vi "Plot Data - Main GUI.vi"() -> ()   [LabVIEW 2017, in "DTacq Plot Display Library.lvlib"]
doc: "This VI is used to display data from the DTacq network enabled drivers.\n\nClicking settings allows the plots on the current tab to be configured."
uses:
  DTacq Plot Display Library.lvlib
  Typedefs/Program Commands--Enum.ctl
  Typedefs/Plot Channel Configruation--Cluster.ctl
  SubVIs/Plot Data--Cluster.ctl
  Network Shared Variables/Typedefs/X and Y Variant Arrays--Cluster.ctl
  Typedefs/Graphical Interface Commands - Tabs--Enum.ctl
  Typedefs/Graphical Interface Commands - Plot--Enum.ctl
  Network Shared Variables/Shared Variables Library.lvlib
panel:
  out "Activity":bool
  out "Last Update":timestamp
  in  "Close Tab Button":bool
  out "XY Plot Title":string
  in  "Add Tab Button":bool
  out "XY Graph":cluster{i32[], i32[]}[](graph)
  in  "Tab Control":T1(tab)
  in  "Save Button":bool
  in  "Settings Button":bool
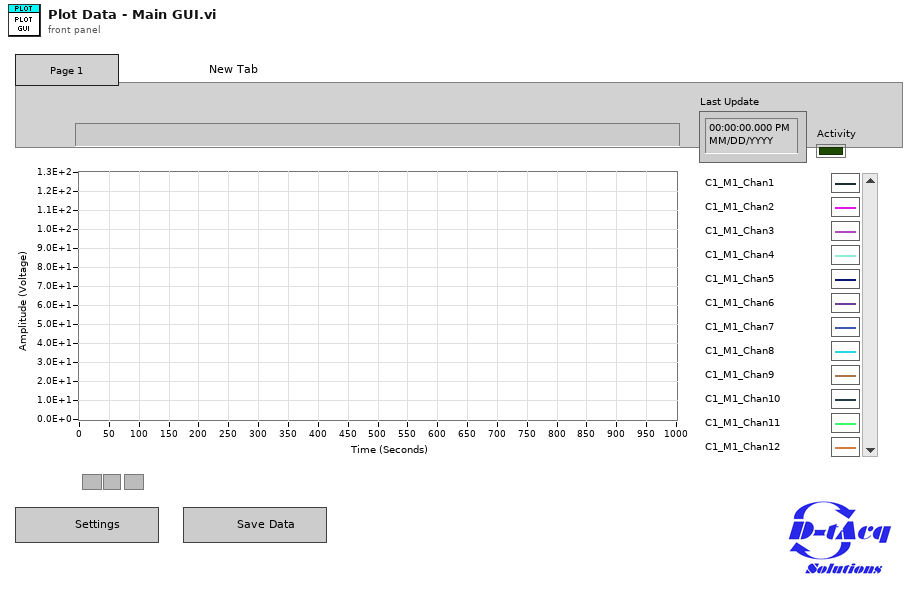
[diagram p1: front panel]
types:
  T1 = enum32{"Page 1", "Page 2", "Page 3", "Page 4", "Page 5", "Page 6"}
  T2 = typedef "DTacq Plot Display Library.lvlib/Plot Data--Cluster.ctl" = cluster{"Last Update":timestamp, "Data Cluster":T3}
  T3 = typedef "Shared Variables Library.lvlib/X and Y Variant Arrays--Cluster.ctl" = cluster{"X-Data":variant[], "Y-Data":variant[]}
  T4 = typedef "DTacq Plot Display Library.lvlib/Plot Channel Configruation--Cluster.ctl" = cluster{"Shared Variable Reference":refnum<k21>, "Full Variable Name":string, "URL":string, "Descriptive Name":string, "Data Type":variant, "Colour":u32}
  T5 = cluster{"Plot Title":string, "Y-Axis Label":string, "X-Axis Label":string, "Plot Channel Configurations":T4[]}
  T6 = typedef "DTacq Plot Display Library.lvlib/Program Commands--Enum.ctl" = enum16{"Save Data", "Read Variable Values", "Set Plot Title", "Open Variable Connections", "Change Settings", "Update Button Positions", "Add Tab", "Close Tab", "Update Plot Display", "Tab Change", "Exit Program", "Update Plot Legend", "User Confirmation", "Load Defaults", "Initialise"}
  T7 = cluster{"Plot Title":string, "Y-Axis Label":string, "X-Axis Label":string, "Plot Channel Configurations":T4[]}[]
  T8 = typedef "DTacq Plot Display Library.lvlib/Graphical Interface Commands - Plot--Enum.ctl" = enum16{"Initialise", "Set Plot Title"}
  T9 = typedef "DTacq Plot Display Library.lvlib/Graphical Interface Commands - Tabs--Enum.ctl" = enum16{"Close GUI", "Initialise", "Add Tab", "Close Tab", "Update Buttons"}
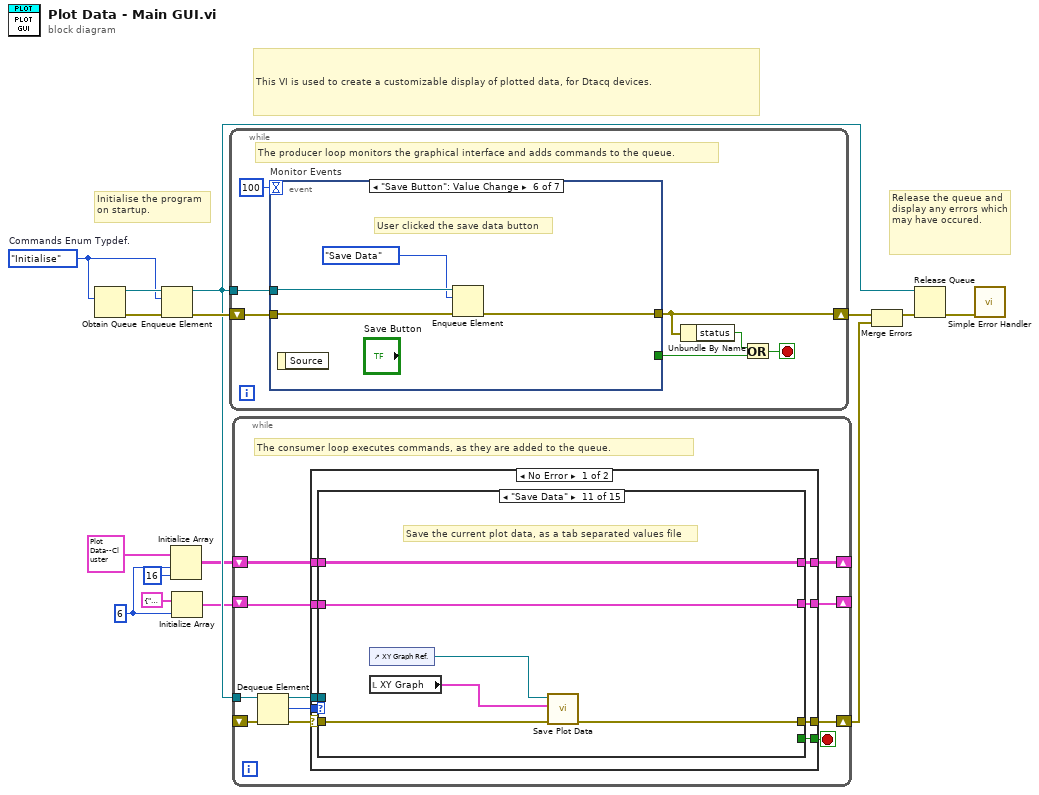
[diagram p0: block diagram]
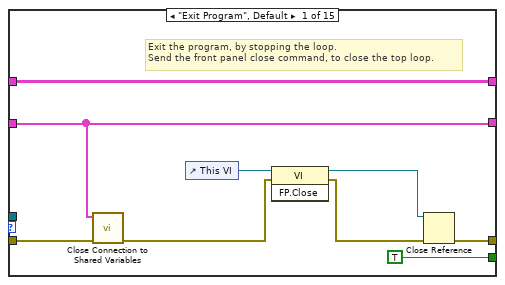
[diagram p2: hidden frame]
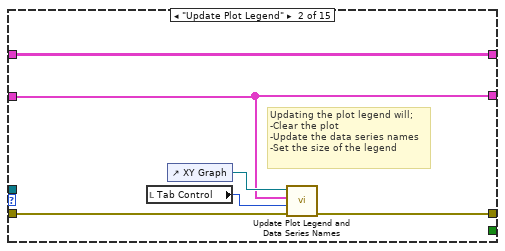
[diagram p3: hidden frame]
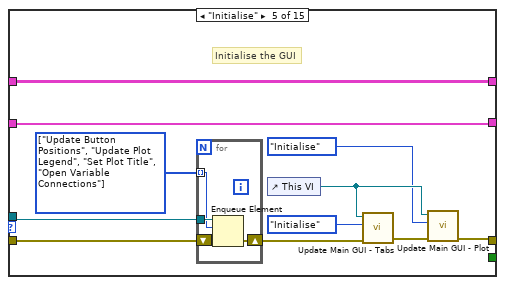
[diagram p6: hidden frame]
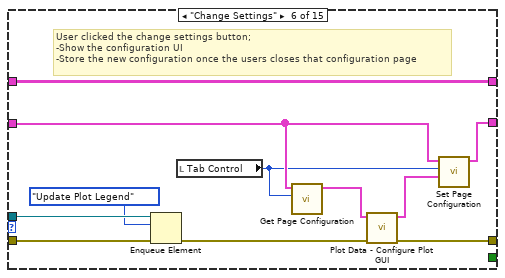
[diagram p7: hidden frame]
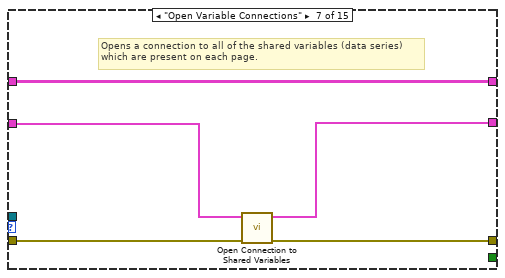
[diagram p8: hidden frame]
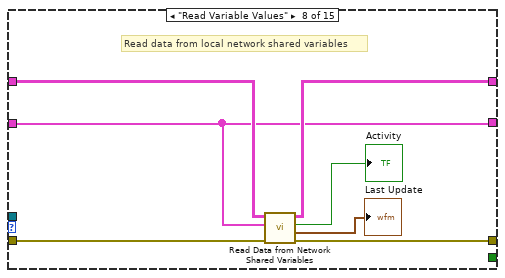
[diagram p9: hidden frame]
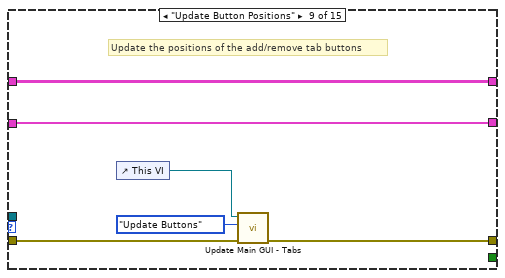
[diagram p10: hidden frame]
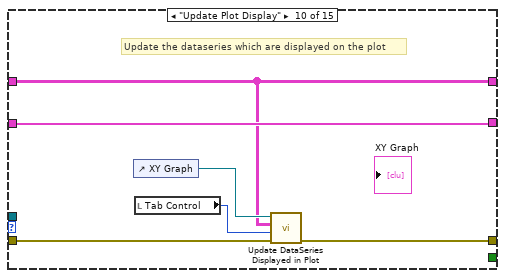
[diagram p11: hidden frame]
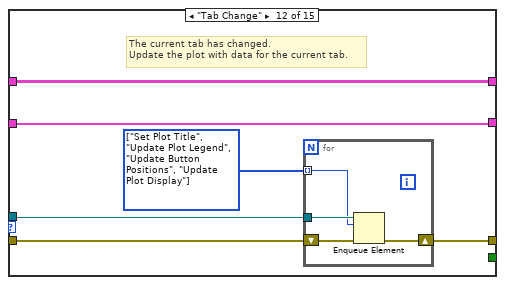
[diagram p12: hidden frame]
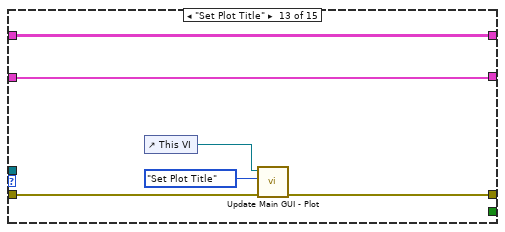
[diagram p13: hidden frame]
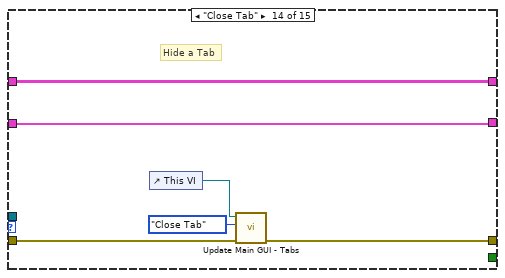
[diagram p14: hidden frame]
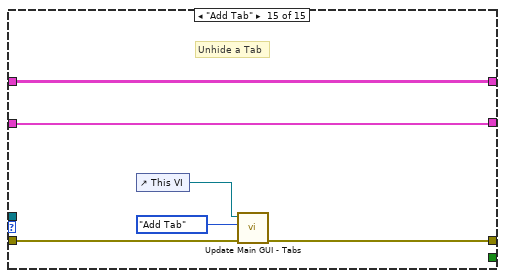
[diagram p15: hidden frame]
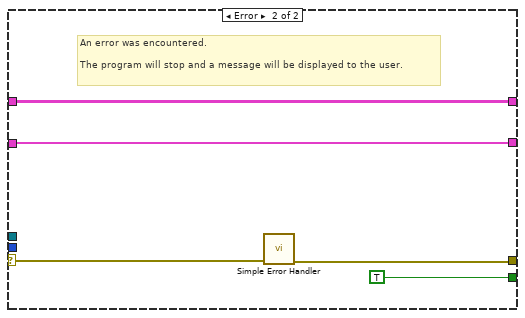
[diagram p16: hidden frame]
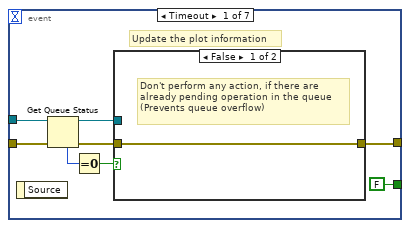
[diagram p17: hidden frame]
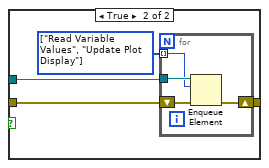
[diagram p18: hidden frame]
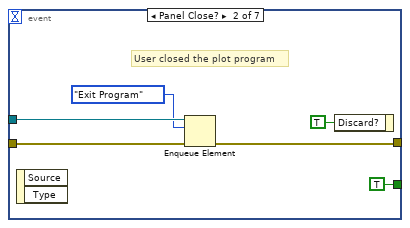
[diagram p19: hidden frame]
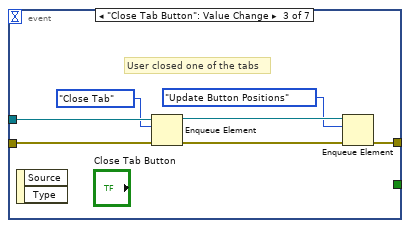
[diagram p20: hidden frame]
diagram:
  w4 = 6 ("dimension size")
  w11 = Program_Commands--Enum."Initialise"  # Commands Enum Typdef.
  # "Initialise the program\non startup."
  # "Release the queue and display any errors which may have occured."
  # "This VI is used to create a customizable display of plotted data, for Dtacq devices."
  n1 = Obtain Queue(element data type=w11) -> (queue out=w15:refnum<queue>, error out=w14:errorcluster)  [unwired: 4 in, 1 out]
  n2 = Enqueue Element(queue=w15, element=w11, error in (no error)=w14) -> (queue out=w12:refnum<queue>, error out=w13:errorcluster)  [unwired: 1 in, 1 out]
  n3 = Initialize Array(T2 {"Last Update"=timestamp(0 s since 1904-01-01), "Data Cluster"={"X-Data"=[], "Y-Data"=[]}}, w4, 16 ("dimension size")) -> (w1:T2[][])
  n4 = Initialize Array(T5 {"Plot Title"="", "Y-Axis Label"="", "X-Axis Label"="", "Plot Channel Configurations"=[]} ("Page Configuration"), w4) -> (w5:T7)
  n5 = while {
    shift-right: [w18] -> w9
    shift-left: w13 -> [w21]
    tunnel: w12 -> [w22]
    stop <- w19 stop-if-true
    # "The producer loop monitors the graphical interface and adds commands to the queue."
    n6 = event "Monitor Events" shown="[5] \"Save Button\": Value Change" {
      selector: _ -> [_ _ _ _ _ _ _]
      dyn-events: _ -> [_ _ _ _ _ _ _]
      timeout: 100 -> [_ _ _ _ _ _ _]
      tunnel: w22 -> [w28 w43 w51 w59 w63 w67 w71]
      tunnel: w21 -> [w27 w44 w52 w58 w64 w68 w72]
      tunnel: [w30 w45 w48 w54 w60 w66 w70] -> w18
      tunnel: [FALSE ("stop") TRUE ("stop") _ _ _ _ _] -> w20
      event Timeout {
        # "Update the plot information"
        n7 = event-data() -> ()  [unwired: 1 in, 1 out]
        n8 = Get Queue Status(queue=w28, error in (no error)=w27) -> (queue out=w26:refnum<queue>, error out=w25:errorcluster, # elements in queue=w24:i32)  [unwired: 1 in, 5 out]
        n9 = Equal To 0?(x=w24) -> (x = 0?=w23:bool)
        n10 = case shown="False" w23 {
          tunnel: [w31 w35] -> w30
          tunnel: w26 -> [_ w33]
          tunnel: w25 -> [w31 w32]
          frame False {
            # "Don't perform any action, if there are\nalready pending operation in the queue\n(Prevents queue overflow)"
          }
          frame True {
            w34 = T6[] [enum."Read Variable Values", enum."Update Plot Display"] items=["Save Data", "Read Variable Values", "Set Plot Title", "Open Variable Connections", "Change Settings", "Update Button Positions", "Add Tab", "Close Tab", "Update Plot Display", "Tab Change", "Exit Program", "Update Plot Legend", "User Confirmation", "Load Defaults", "Initialise"] ("appended array")
            n11 = for {
              tunnel: w33 -> [w38]
              shift-right: [w37] -> w35
              shift-left: w32 -> [w39]
              tunnel: w34 -> [w36] mode=indexing
              n12 = Enqueue Element(queue=w38, element=w36, error in (no error)=w39) -> (error out=w37:errorcluster)  [unwired: 1 in, 2 out]
            }
          }
        }
      }
      event Panel Close? {
        # "User closed the plot program"
        n13 = event-data() -> ()  [unwired: 1 in, 2 out]
        n14 = Enqueue Element(queue=w43, element=Program_Commands--Enum."Exit Program", error in (no error)=w44) -> (error out=w45:errorcluster)  [unwired: 1 in, 2 out]
        n15 = event-data("Discard?"=TRUE) -> ()  [unwired: 1 in, 1 out]
      }
      event "Close Tab Button": Value Change {
        # "User closed one of the tabs"
        n16 = event-data() -> ()  [unwired: 1 in, 2 out]
        n17 = Enqueue Element(queue=w51, element=Program_Commands--Enum."Close Tab", error in (no error)=w52) -> (queue out=w47:refnum<queue>, error out=w49:errorcluster)  [unwired: 1 in, 1 out]
        n18 = Enqueue Element(queue=w47, element=Program_Commands--Enum."Update Button Positions", error in (no error)=w49) -> (error out=w48:errorcluster)  [unwired: 1 in, 2 out]
      }
      event "Add Tab Button": Value Change {
        # "User clicked the add tab button"
        n19 = event-data() -> ()  [unwired: 1 in, 2 out]
        n20 = Enqueue Element(queue=w59, element=Program_Commands--Enum."Add Tab", error in (no error)=w58) -> (queue out=w55:refnum<queue>, error out=w56:errorcluster)  [unwired: 1 in, 1 out]
        n21 = Enqueue Element(queue=w55, element=Program_Commands--Enum."Update Button Positions", error in (no error)=w56) -> (error out=w54:errorcluster)  [unwired: 1 in, 2 out]
      }
      event "Tab Control": Value Change {
        # "User changed the current tab"
        n22 = event-data() -> ()  [unwired: 1 in, 1 out]
        n23 = local write "Tab Control"("Tab Control") -> ()
        n24 = Enqueue Element(queue=w63, element=Program_Commands--Enum."Tab Change", error in (no error)=w64) -> (error out=w60:errorcluster)  [unwired: 1 in, 2 out]
      }
      event "Save Button": Value Change {
        # "User clicked the save data button"
        n25 = event-data() -> ()  [unwired: 1 in, 1 out]
        n26 = Enqueue Element(queue=w67, element=Program_Commands--Enum."Save Data", error in (no error)=w68) -> (error out=w66:errorcluster)  [unwired: 1 in, 2 out]
      }
      event "Settings Button": Value Change {
        # "User clicked the change settings button."
        n27 = event-data() -> ()  [unwired: 1 in, 1 out]
        n28 = Enqueue Element(queue=w71, element=Program_Commands--Enum."Change Settings", error in (no error)=w72) -> (error out=w70:errorcluster)  [unwired: 1 in, 2 out]
      }
    }
    n29 = Unbundle By Name(w18) -> ("status"=w17:bool)
    n30 = Or(x=w17, y=w20) -> (x .or. y?=w19:bool)
  }
  n31 = while {
    tunnel: w12 -> [w83]
    shift-right: [w79] -> w10
    shift-left: _ -> [w78]
    shift-right: [w75] -> _
    shift-left: w5 -> [w76]
    shift-right: [w73] -> _
    shift-left: w1 -> [w74]
    stop <- w80 stop-if-true
    # "The consumer loop executes commands, as they are added to the queue."
    n32 = Dequeue Element(queue=w83, error in (no error)=w78) -> (queue out=w77:refnum<queue>, element=w81:T6, error out=w82:errorcluster)  [unwired: 1 in, 1 out]
    n33 = case shown="No Error" w82 {
      selector: w82 -> [w91 w199]
      tunnel: w81 -> [w92 _]
      tunnel: [w89 TRUE] -> w80
      tunnel: [w90 w198] -> w79
      tunnel: w77 -> [w88 _]
      tunnel: w76 -> [w87 w201]
      tunnel: [w86 w201] -> w75
      tunnel: w74 -> [w85 w200]
      tunnel: [w84 w200] -> w73
      frame No Error {
        n34 = case shown="\"Save Data\"" w92 {
          tunnel: w91 -> [w95 w103 w110 w113 w124 w133 w143 w147 w156 w160 w165 w173 w181 w190 w196]
          tunnel: [w98 w104 w110 w113 w119 w139 w142 w150 w157 w159 w164 w172 w180 w191 w197] -> w90
          tunnel: [TRUE _ _ _ _ _ _ _ _ _ _ _ _ _ _] -> w89
          tunnel: w88 -> [_ _ _ _ w123 w131 _ _ _ _ _ w171 _ _ _]
          tunnel: w87 -> [w93 w106 w109 w112 w116 w136 w144 w148 w153 w163 w169 w175 w185 w187 w193]
          tunnel: [w93 w106 w109 w112 w116 w134 w141 w148 w153 w163 w169 w175 w185 w187 w193] -> w86
          tunnel: w85 -> [w100 w102 w108 w111 w115 w129 w140 w149 w152 w158 w168 w174 w184 w186 w192]
          tunnel: [w100 w102 w108 w111 w115 w129 w140 w151 w152 w158 w168 w174 w184 w186 w192] -> w84
          frame "Exit Program", Default {
            # "Exit the program, by stopping the loop.\nSend the front panel close command, to close the top loop."
            n35 = call "Close Connection to Shared Variables.vi"("Error In"=w95, "Page Configurations In"=w93) -> ("Error Out"=w94:errorcluster)  [unwired: 8 in, 1 out]
            n36 = control-ref of="This VI"() -> (w99:refnum<vi>)
            n37 = invoke class="VI" method="FP.Close"(reference=w99, error in=w94) -> (reference out=w96:refnum<vi>, error out=w97:errorcluster)  [unwired: 1 in, 1 out]
            n38 = Close Reference(reference=w96, error in (no error)=w97) -> (error out=w98:errorcluster)
          }
          frame "Update Plot Legend" {
            # "Updating the plot legend will;\n-Clear the plot\n-Update the data series names\n-Set the size of the legend"
            n39 = local read "Tab Control"() -> (w105:T1)
            n40 = control-ref of="XY Graph"() -> (w107:refnum<vi>)
            n41 = call "Update Plot Legend and Data Series Names.vi"("error in"=w103, "Active Tab"=w105, "Page Configurations In"=w106, "XYGraph Ref In"=w107) -> ("error out"=w104:errorcluster)  [unwired: 7 in]
          }
          frame "User Confirmation" {
          }
          frame "Load Defaults" {
          }
          frame "Initialise" {
            w114 = T6[] [enum."Update Button Positions", enum."Update Plot Legend", enum."Set Plot Title", enum."Open Variable Connections"] items=["Save Data", "Read Variable Values", "Set Plot Title", "Open Variable Connections", "Change Settings", "Update Button Positions", "Add Tab", "Close Tab", "Update Plot Display", "Tab Change", "Exit Program", "Update Plot Legend", "User Confirmation", "Load Defaults", "Initialise"] ("appended array")
            # "Initialise the GUI"
            n42 = for {
              tunnel: w123 -> [w127]
              shift-right: [w126] -> w122
              shift-left: w124 -> [w128]
              tunnel: w114 -> [w125] mode=indexing
              n43 = Enqueue Element(queue=w127, element=w125, error in (no error)=w128) -> (error out=w126:errorcluster)  [unwired: 1 in, 2 out]
            }
            n44 = control-ref of="This VI"() -> (w118:refnum<vi>)
            n45 = call "Update Main GUI - Tabs.vi"("error in"=w122, "GUI Command"=Graphical_Interface_Commands_-_Tabs--Enum."Initialise", "Main GUI Refnum"=w118) -> ("error out"=w120:errorcluster)  [unwired: 8 in]
            n46 = call "Update Main GUI - Plot.vi"("error in"=w120, "GUI Command"=Graphical_Interface_Commands_-_Plot--Enum."Initialise", "Main GUI Refnum"=w118) -> ("error out"=w119:errorcluster)  [unwired: 8 in]
          }
          frame "Change Settings" {
            # "User clicked the change settings button;\n-Show the configuration UI\n-Store the new configuration once the users closes that configuration page"
            n47 = Enqueue Element(queue=w131, element=Program_Commands--Enum."Update Plot Legend", error in (no error)=w133) -> (error out=w132:errorcluster)  [unwired: 1 in, 2 out]
            n48 = local read "Tab Control"() -> (w135:T1)
            n49 = call "Get Page Configuration.vi"("Page Number"=w135, "Page Configurations"=w136) -> ("Plot Channel Configurations"=w138:T4[])  [unwired: 9 in]
            n50 = call "Plot Data - Configure Plot GUI.vi"("Error In"=w132, "Plot Channel Configurations In"=w138) -> ("Error Out"=w139:errorcluster, "Plot Channel Configurations Out"=w137:T4[])  [unwired: 8 in]
            n51 = call "Set Page Configuration.vi"("Plot Channel Configurations"=w137, "Page Number"=w135, "Page Configurations In"=w136) -> ("Page Configurations Out"=w134:T7)  [unwired: 8 in]
          }
          frame "Open Variable Connections" {
            # "Opens a connection to all of the shared variables (data series)\nwhich are present on each page."
            n52 = call "Open Connection to Shared Variables.vi"("Error In"=w143, "Page Configurations In"=w144) -> ("Error Out"=w142:errorcluster, "Page Configurations Out"=w141:T7)  [unwired: 8 in]
          }
          frame "Read Variable Values" {
            # "Read data from local network shared variables"
            n53 = call "Read Data from Network Shared Variables.vi"("error in"=w147, "Page Configurations"=w148, "Plot Data In"=w149) -> ("error out"=w150:errorcluster, "Update Time"=→"Last Update":timestamp, "New Data"=→"Activity":bool, "Plot Data Out"=w151:T2[][])  [unwired: 5 in]
          }
          frame "Update Button Positions" {
            # "Update the positions of the add/remove tab buttons"
            n54 = control-ref of="This VI"() -> (w155:refnum<vi>)
            n55 = call "Update Main GUI - Tabs.vi"("error in"=w156, "GUI Command"=Graphical_Interface_Commands_-_Tabs--Enum."Update Buttons", "Main GUI Refnum"=w155) -> ("error out"=w157:errorcluster)  [unwired: 8 in]
          }
          frame "Update Plot Display" {
            # "Update the dataseries which are displayed on the plot"
            n56 = control-ref of="XY Graph"() -> (w161:refnum<vi>)
            n57 = local read "Tab Control"() -> (w162:T1)
            n58 = call "Update DataSeries Displayed in Plot.vi"("error in"=w160, "Tab Control"=w162, "Plot Data"=w158, "XYGraph Ref In"=w161) -> ("error out"=w159:errorcluster)  [unwired: 7 in]
          }
          frame "Save Data" {
            # "Save the current plot data, as a tab separated values file"
            n59 = control-ref of="XY Graph Ref."() -> (w166:refnum<vi>)
            n60 = local read "XY Graph"() -> (w167:cluster{i32[], i32[]}[])
            n61 = call "Save Plot Data.vi"("error in"=w165, "XY Graph"=w167, "XYGraph in"=w166) -> ("error out"=w164:errorcluster)  [unwired: 8 in]
          }
          frame "Tab Change" {
            w170 = T6[] [enum."Set Plot Title", enum."Update Plot Legend", enum."Update Button Positions", enum."Update Plot Display"] items=["Save Data", "Read Variable Values", "Set Plot Title", "Open Variable Connections", "Change Settings", "Update Button Positions", "Add Tab", "Close Tab", "Update Plot Display", "Tab Change", "Exit Program", "Update Plot Legend", "User Confirmation", "Load Defaults", "Initialise"] ("appended array")
            # "The current tab has changed.\nUpdate the plot with data for the current tab."
            n62 = for {
              tunnel: w171 -> [w177]
              shift-right: [w178] -> w172
              shift-left: w173 -> [w179]
              tunnel: w170 -> [w176] mode=indexing
              n63 = Enqueue Element(queue=w177, element=w176, error in (no error)=w179) -> (error out=w178:errorcluster)  [unwired: 1 in, 2 out]
            }
          }
          frame "Set Plot Title" {
            n64 = control-ref of="This VI"() -> (w183:refnum<vi>)
            n65 = call "Update Main GUI - Plot.vi"("error in"=w181, "GUI Command"=Graphical_Interface_Commands_-_Plot--Enum."Set Plot Title", "Main GUI Refnum"=w183) -> ("error out"=w180:errorcluster)  [unwired: 8 in]
          }
          frame "Close Tab" {
            # "Hide a Tab"
            n66 = control-ref of="This VI"() -> (w189:refnum<vi>)
            n67 = call "Update Main GUI - Tabs.vi"("error in"=w190, "GUI Command"=Graphical_Interface_Commands_-_Tabs--Enum."Close Tab", "Main GUI Refnum"=w189) -> ("error out"=w191:errorcluster)  [unwired: 8 in]
          }
          frame "Add Tab" {
            # "Unhide a Tab"
            n68 = control-ref of="This VI"() -> (w195:refnum<vi>)
            n69 = call "Update Main GUI - Tabs.vi"("error in"=w196, "GUI Command"=Graphical_Interface_Commands_-_Tabs--Enum."Add Tab", "Main GUI Refnum"=w195) -> ("error out"=w197:errorcluster)  [unwired: 8 in]
          }
        }
      }
      frame Error {
        # "An error was encountered.\n\nThe program will stop and a message will be displayed to the user."
        n70 = call <vilib>:"Simple Error Handler.vi"("error in (no error)"=w199) -> ("error out"=w198:errorcluster)  [unwired: 4 in, 4 out]
      }
    }
  }
  n71 = Merge Errors(w9, w10) -> (w8:errorcluster)
  n72 = Release Queue(queue=w12, error in (no error)=w8) -> (error out=w7:errorcluster)  [unwired: 1 in, 2 out]
  n73 = call <vilib>:"Simple Error Handler.vi"("error in (no error)"=w7) -> ()  [unwired: 4 in, 5 out]
